vi "Request Logger.vi"(8 "error in (no error)":errorcluster, 11 "Log Producer in":T1) -> (0 "error out":errorcluster, 3 "Log Producer out":T1)   [LabVIEW 2020, in "Frame Logging.lvlib"]
uses:
  Frame Logging.lvlib
  Log_Producer.ctl
  Message_Request.ctl
  Message_Request_Action.ctl
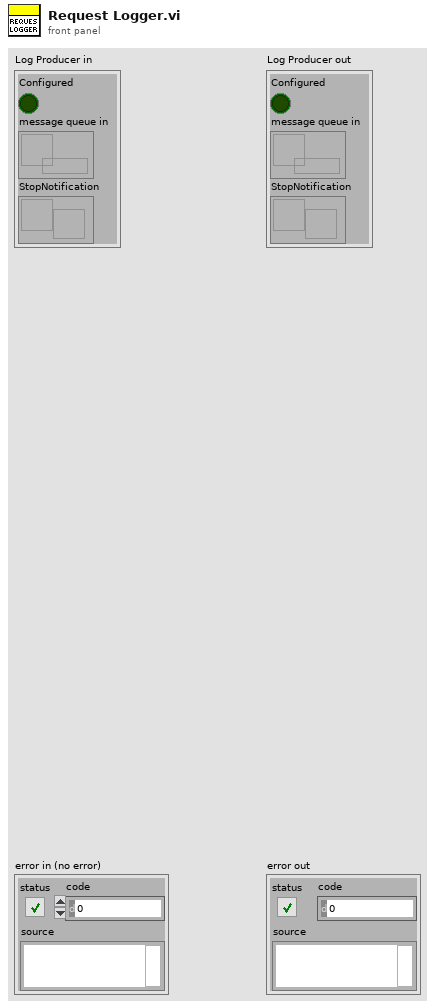
[diagram p1: front panel]
types:
  T1 = typedef "Frame Logging.lvlib/Log_Producer.ctl" = cluster{"Configured":bool, "message queue in":refnum<queue>, "StopNotification":refnum<notifier>}
  T2 = typedef "Frame Logging.lvlib/Message_Request.ctl" = cluster{"request":T3, "data":variant}
  T3 = typedef "Frame Logging.lvlib/Message_Request_Action.ctl" = enum16{"Initialize", "Open File", "Log", "Manage Disk", "Stop", "Close File", "Update Configuration"}
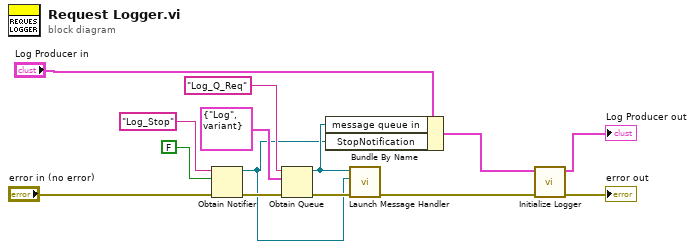
[diagram p0: block diagram]
diagram:
  n1 = Obtain Notifier(name (unnamed)="Log_Stop", notification data type=FALSE, error in (no error)="error in (no error)") -> (notifier out=w5:refnum<notifier>, error out=w8:errorcluster)  [unwired: 1 in, 1 out]
  n2 = Obtain Queue(name (unnamed)="Log_Q_Req", element data type=T2 {"request"=enum."Log", "data"=variant} ("Message_type"), error in (no error)=w8) -> (queue out=w12:refnum<queue>, error out=w11:errorcluster)  [unwired: 2 in, 1 out]
  n3 = Bundle By Name(cluster="Log Producer in", "message queue in"=w12, "StopNotification"=w5) -> (w3:T1)
  n4 = call "Launch Message Handler.vi"("error in (no error)"=w11, "stop notifier"=w5, "message queue in"=w12) -> ("error out"=w4:errorcluster)  [unwired: 8 in]
  n5 = call "Initialize Logger.vi"("error in"=w4, "Log Producer in"=w3) -> ("error out"=→"error out":errorcluster, "Log Producer out"=→"Log Producer out":T1)  [unwired: 8 in]
